vi "RT_DETR_OpenVINO_imgs.vi"() -> ()   [LabVIEW 2018]
doc: "(2)RT-DETR_OpenVINO_imgs: This example is an object detection example of the RT-DETR algorithm, which can achieve object detection function on sample images."
uses:
  vi.lib/VIRobotics/opencv_yiku/Mat/Mat_8U/Mat_8U.lvclass
  C:/nuc/.package/vi.lib/VIRobotics/opencv_yiku/Mat/Mat/Mat.lvclass
  vi.lib/VIRobotics/ModelZoo/Object_Detection/RT_DETR_OpenVINO/InitialModel_RT_DETR_OpenVINO.vi
  vi.lib/VIRobotics/opencv_yiku/Mat/Mat/Mat_release.vi
  vi.lib/VIRobotics/ModelZoo/Object_Detection/RT_DETR_OpenVINO/RT_DETR_OpenVINO.lvclass
  vi.lib/VIRobotics/opencv_yiku/opencv_yiku.lvlib
  vi.lib/VIRobotics/opencv_yiku/Mat/Mat/Mat.lvclass
panel:
  in  "device_name":string(combo)="CPU"
  out "每帧耗时(s)":dbl
  in  "model_file":path=path "C:/ProgramData/VIRobotics/ModelZoo/Object_Detection/RT_DETR/onnx_model/rtdetr_r50vd_m_6x_coco.onnx"
  in  "class_names_file":path=path "C:/ProgramData/VIRobotics/ModelZoo/Object_Detection/coco.names"
  out "picture":picture
  in  "imgs":i32(listbox)=1
  in  "image Folder":path=path "C:/ProgramData/VIRobotics/ModelZoo/Object_Detection/imgs"
  in  "stop":bool
  # "Overview: Demonstrates how to read a collection of images and use OpenVINO to load the ONNX model of pp-rtdetr for object detection.\nRequirements: Windows.\nInstructions: \nIf you want to load the model, follow the following steps:\n1.Select the device_name to use. \n2.Specify the model_file and class_names_file(Because the model is too large, it is not loaded by default.).\n3.Run the VI.\n4.Specify the path of the image Folder and click on the image in the imgs control on the right side of the interface that need to be detected."
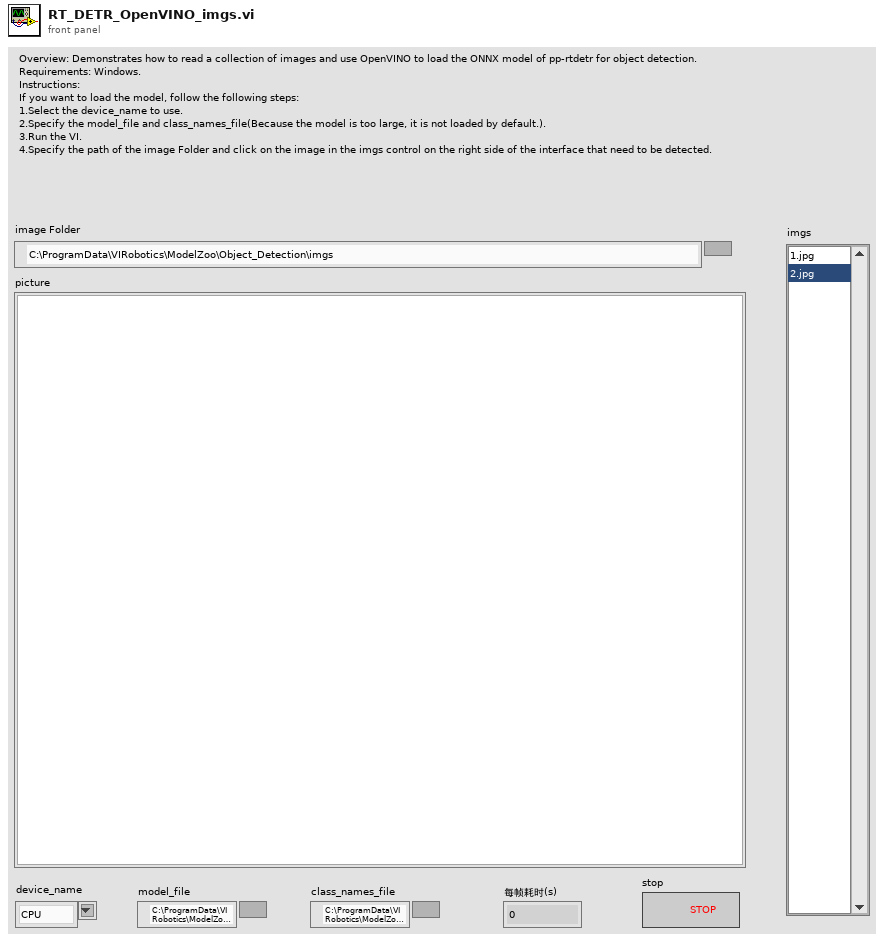
[diagram p1: front panel]
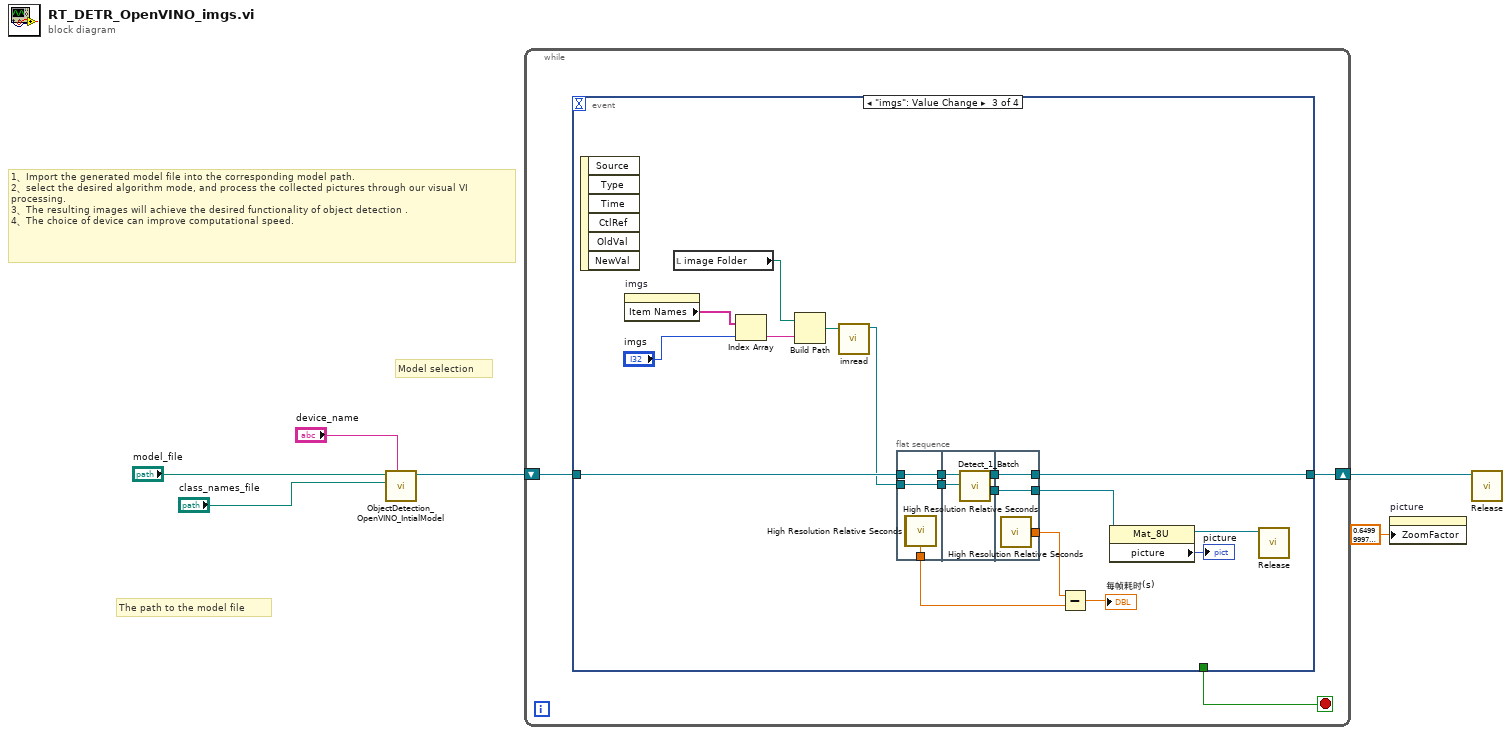
[diagram p0: block diagram]
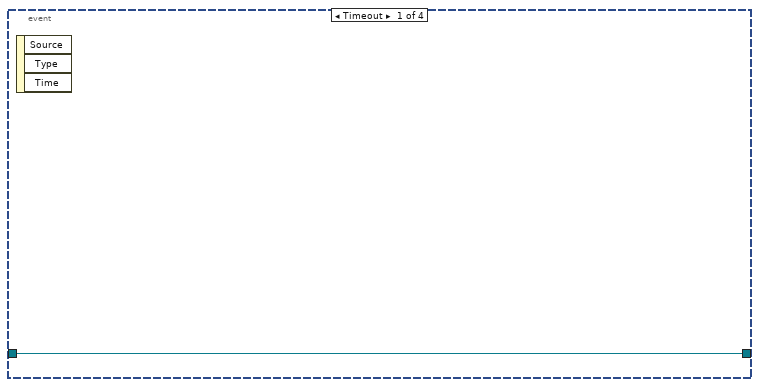
[diagram p2: hidden frame]
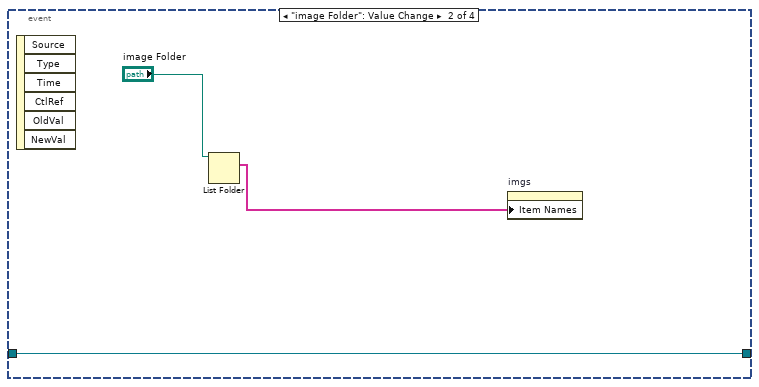
[diagram p3: hidden frame]
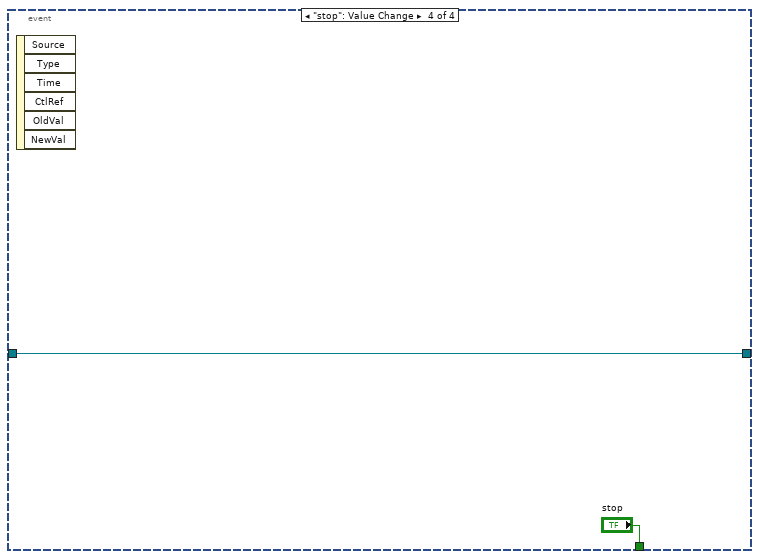
[diagram p4: hidden frame]
diagram:
  # "1、Import the generated model file into the corresponding model path. \n2、select the desired algorithm mode, and process the collected pictures through our visual VI processing. \n3、The resulting images will achieve the desired functionality of object detection . \n4、The choice of device can improve computational speed."
  # "Model selection"
  # "The path to the model file"
  n1 = call-poly "ObjectDetection_OpenVINO_IntialModel.vi"("device_name"="device_name", "class_names_path"="class_names_file", "onnx_file"="model_file") -> ("detr_ov out"=w5:refnum<class "RT_DETR_OpenVINO.lvclass">)  [unwired: 7 in, 1 out]
  n2 = while {
    shift-right: [w8] -> w6
    shift-left: w5 -> [w9]
    stop <- w7 stop-if-true
    n3 = event shown="[2] \"imgs\": Value Change" {
      selector: _ -> [_ _ _ _]
      dyn-events: _ -> [_ _ _ _]
      timeout: _ -> [_ _ _ _]
      tunnel: w9 -> [w10 w11 w26 w42]
      tunnel: [w10 w11 w25 w42] -> w8
      tunnel: [_ _ _ "stop"] -> w7
      event Timeout {
        n4 = event-data() -> ()  [unwired: 1 in, 3 out]
      }
      event "image Folder": Value Change {
        n5 = event-data() -> ()  [unwired: 1 in, 6 out]
        n6 = List Folder(path="image Folder") -> (filenames=w12:string[])  [unwired: 3 in, 3 out]
        n7 = property on="imgs" class="LstBox (strict)"("Item Names"=w12) -> ()  [unwired: 2 in, 2 out]
      }
      event "imgs": Value Change {
        n8 = event-data() -> ()  [unwired: 1 in, 6 out]
        n9 = property on="imgs" class="LstBox (strict)"() -> ("Item Names"=w31:string[])  [unwired: 2 in, 2 out]
        n10 = local read "image Folder"() -> (w28:path)
        n11 = Index Array(array=w31, index="imgs") -> (element=w29:string)
        n12 = Build Path(base path=w28, name or relative path=w29) -> (appended path=w27:path)
        n13 = call "imread.vi"("path"=w27) -> ("Mat out"=w15:refnum<class "Mat_8U.lvclass">)  [unwired: 9 in, 1 out]
        n14 = flat-sequence {
          tunnel: w26 -> [w34]
          tunnel: [w34] -> w21
          tunnel: [w33] -> w17
          tunnel: w15 -> [w32]
          tunnel: [w32] -> w14
          tunnel: w21 -> [w38]
          tunnel: [w37] -> w20
          tunnel: [w36] -> w19
          tunnel: w14 -> [w35]
          tunnel: [w40] -> w24
          tunnel: [w41] -> w25
          tunnel: w20 -> [w41]
          tunnel: w19 -> [w40]
          tunnel: [w39] -> w18
          frame #0 {
            n15 = call <vilib>:"High Resolution Relative Seconds.vi"() -> ("relative seconds"=w33:dbl)
            n16 = call <vilib>:"High Resolution Relative Seconds.vi"() -> ()  [unwired: 1 out]
          }
          frame #1 {
            n17 = call-dynamic "Detect_1_Batch.vi"("image"=w35, "RT_DETR_OpenVINO in"=w38) -> ("img out"=w36:refnum<class "Mat_8U.lvclass">, "RT_DETR_OpenVINO out"=w37:refnum<class "RT_DETR_OpenVINO.lvclass">)  [unwired: 6 in, 2 out]
          }
          frame #2 {
            n18 = call <vilib>:"High Resolution Relative Seconds.vi"() -> ("relative seconds"=w39:dbl)
          }
        }
        n19 = Subtract(x=w18, y=w17) -> (x-y=→"每帧耗时(s)":dbl)
        n20 = property class="Mat_8U"(reference=w24) -> (reference out=w22:refnum<class "Mat_8U.lvclass">, "picture"=→"picture":picture)  [unwired: 1 in, 1 out]
        n21 = call-poly "Release.vi"("Mat in"=w22) -> ()  [unwired: 10 in, 1 out]
      }
      event "stop": Value Change {
        n22 = event-data() -> ()  [unwired: 1 in, 6 out]
      }
    }
  }
  n23 = property on="picture" class="Pict"("ZoomFactor"=sgl 0.65 ("Zoom Factor")) -> ()  [unwired: 2 in, 2 out]
  n24 = call-dynamic "Release.vi"("RT_DETR_OpenVINO in"=w6) -> ()  [unwired: 9 in, 2 out]
